vi "Auto_Zoom_Limelight.vi"(1 "Target_Horizontal Angle":dbl, 2 "Verticle_Angle":dbl, 3 "Is_Target_Visible?":bool) -> (0 "Zoom_Indicator":T1=enum."Zoom2x")   [LabVIEW 2019]
uses:
  ArgosLib/ArgosLib.lvlib
  Vision/TypeDefs/VisionPipeline.ctl
  ArgosLib/Signal Processing/TypeDefs/Hysteresis_State.ctl
panel:
  in  "Horizontal_Zoom_HYS_Range":dbl
  in  "Horizontal_FOV_Angle":dbl
  in  "Target_Visible_Debounce_Time (MS)":u32
  in  "Verticle_Zoom_HYS_Range":dbl
  in  "Vertical_FOV_Angle":dbl
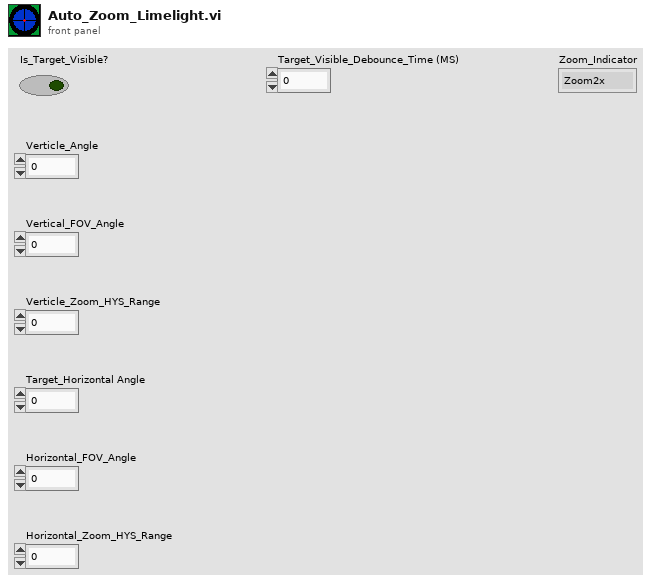
[diagram p1: front panel]
types:
  T1 = typedef "VisionPipeline.ctl" = enum16{"LEDOff", "NoZoom", "Zoom2x", "Zoom3x"}
  T2 = typedef "Hysteresis_State.ctl" = enum16{"Above Threshold", "Below Threshold"}
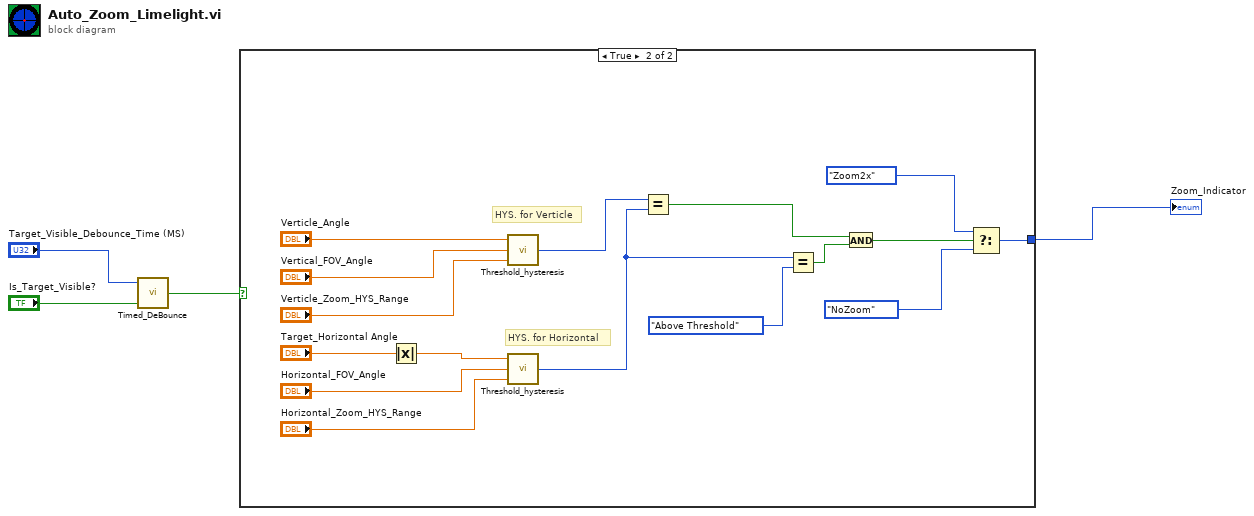
[diagram p0: block diagram]
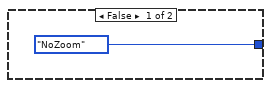
[diagram p2: hidden frame]
diagram:
  n1 = call "Timed_DeBounce.vi"("Input"="Is_Target_Visible?", "Hold Time(ms)"="Target_Visible_Debounce_Time (MS)") -> ("Output"=w4:bool)  [unwired: 1 in]
  n2 = case shown="True" w4 {
    tunnel: [VisionPipeline."NoZoom" ("Enum") w13] -> w1
    frame False {
    }
    frame True {
      # "HYS. for Horizontal"
      # "HYS. for Verticle"
      n3 = Absolute Value(x="Target_Horizontal Angle") -> (abs(x)=w6:dbl)
      n4 = call "Threshold_hysteresis.vi"("Range"="Verticle_Zoom_HYS_Range", "Threshold"="Vertical_FOV_Angle", "X"="Verticle_Angle") -> ("Threshold_State"=w8:T2)
      n5 = call "Threshold_hysteresis.vi"("Range"="Horizontal_Zoom_HYS_Range", "Threshold"="Horizontal_FOV_Angle", "X"=w6) -> ("Threshold_State"=w7:T2)
      n6 = Equal?(x=w8, y=w7) -> (x = y?=w15:bool)
      n7 = Equal?(x=w7, y=Hysteresis_State."Above Threshold" ("Threshold_State")) -> (x = y?=w14:bool)
      n8 = And(x=w15, y=w14) -> (x .and. y?=w11:bool)
      n9 = Select(t=VisionPipeline."Zoom2x", s=w11, f=VisionPipeline."NoZoom" ("Enum")) -> (s? t:f=w13:T1)
    }
  }
  "Zoom_Indicator" <- w1
